vi "UpdateLoadCell.vi"(8 "Steps":i8, 9 "Address":i32, 10 "Code67Memory":refnum<k21>, 11 "Code66Memory":refnum<k21>) -> ()   [LabVIEW 2016, in "FPGAMockMDILC.lvlib"]
uses:
  FPGAMockMDILC.lvlib
  <vilib>/rvi/Emulation/niFpgaSctlEmulationGetInTimedLoop.vi
  <vilib>/Utility/error.llb/Clear Errors.vi
  <vilib>/rvi/DataTransferAndStorage/Container/Common/niFpgaContainerExecOnDevCompGetState.vi
  <vilib>/rvi/Emulation/niFpgaEmulationIsFPGAContextNoSignature.vi
  <vilib>/rvi/DataTransferAndStorage/Container/Common/niFpgaContainerGetUniqueNameForEmu.vi
  <vilib>/rvi/Emulation/niFpgaProcessEmulError.vi
  <vilib>/rvi/errors/nirviReportUnexpectedCaseInternalError (U32).vi
  <vilib>/rvi/Memory/Memory_Emulation/niFpgaMemoryEmulationCacheClearOnFirstRun.vi
  <vilib>/rvi/Memory/Memory_Emulation/nirvimemoryEmulationManagerCache_MakeExclusive.vi
  <vilib>/rvi/Memory/Memory_Emulation/niFpgaMemoryEmulationValidateCache.vi
  <vilib>/rvi/Memory/Memory_Emulation/nirvimemoryEmulationManagerCache_InsertValue.vi
  <vilib>/rvi/Memory/Memory_Emulation/nirvimemoryEmulationManagerCache_ReleaseExclusive.vi
  <vilib>/rvi/Memory/Memory_Emulation/nirvimemoryEmulationManagerCache_GetValue.vi
  <vilib>/rvi/Memory/Memory_Emulation/nirvimemoryEmulationManagerCache_SetValue.vi
  <vilib>/rvi/Emulation/niFpgaSctlEmulationResourceMgr.vi
  <vilib>/rvi/DataTransferAndStorage/Container/XNode/niFpgaContainer.xnode
  <vilib>/rvi/Memory/Memory_Emulation/niFpgaMemoryEmulationRefIn.vi
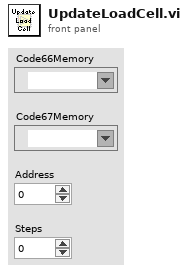
[diagram p1: front panel]
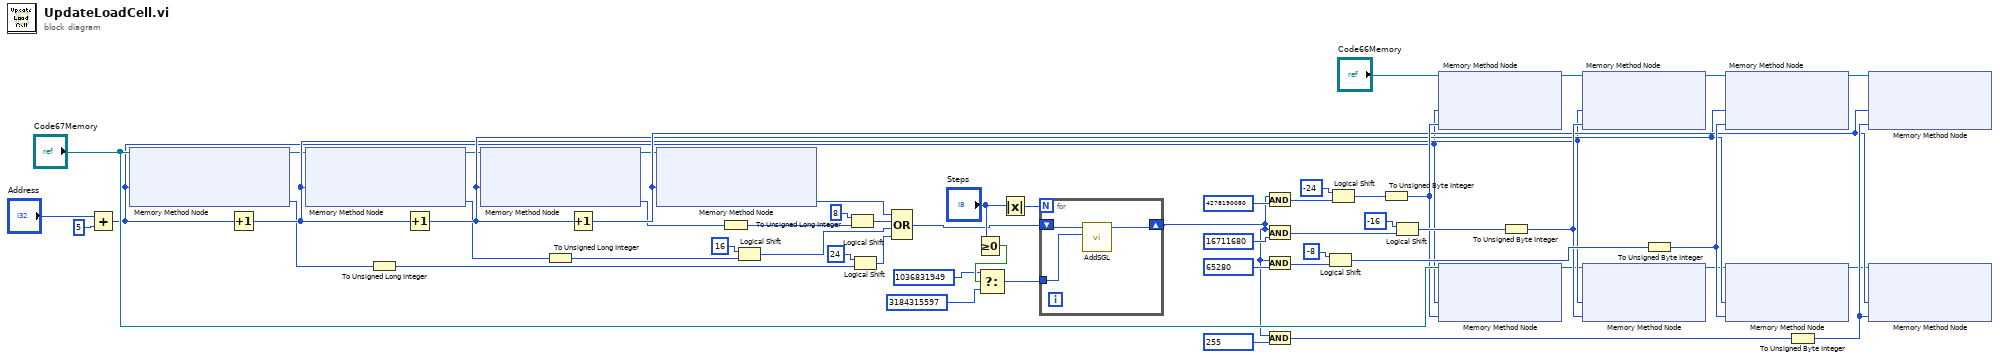
[diagram p0: block diagram]
diagram:
  n1 = Add(x="Address", y=5) -> (x+y=w41:i32)
  n2 = xnode ("Memory Method Node")("Address"=w41, "Memory In"="Code67Memory") -> ("Data"=w12:u8, "Memory Out"=w9:refnum<k21>)
  n3 = Increment(x=w41) -> (x+1=w43:i32)
  n4 = xnode ("Memory Method Node")("Address"=w43, "Memory In"=w9) -> ("Data"=w17:u8, "Memory Out"=w21:refnum<k21>)
  n5 = To Unsigned Long Integer(number=w12) -> (unsigned 32bit integer=w13:u32)
  n6 = Increment(x=w43) -> (x+1=w45:i32)
  n7 = xnode ("Memory Method Node")("Address"=w45, "Memory In"=w21) -> ("Data"=w20:u8, "Memory Out"=w22:refnum<k21>)
  n8 = To Unsigned Long Integer(number=w17) -> (unsigned 32bit integer=w16:u32)
  n9 = Increment(x=w45) -> (x+1=w47:i32)
  n10 = xnode ("Memory Method Node")("Address"=w47, "Memory In"=w22) -> ("Data"=w26:u8)  [unwired: 1 out]
  n11 = To Unsigned Long Integer(number=w20) -> (unsigned 32bit integer=w18:u32)
  n12 = Logical Shift(y=i16 16, x=w16) -> (x << y=w24:u32)
  n13 = Logical Shift(y=i16 8, x=w18) -> (x << y=w25:u32)
  n14 = Logical Shift(y=i16 24, x=w13) -> (x << y=w23:u32)
  n15 = Compound Arithmetic op=OR(w26, w25, w24, w23) -> (w2:u32)
  n16 = Greater Or Equal To 0?(x="Steps") -> (x >= 0?=w6:bool)
  n17 = Select(t=u32 1036831949, s=w6, f=u32 3184315597) -> (s? t:f=w3:u32)
  n18 = Absolute Value(x="Steps") -> (abs(x)=w8:i8)
  n19 = for {
    N: w8 -> [_]
    tunnel: w3 -> [w59]
    shift-right: [w57] -> w1
    shift-left: w2 -> [w58]
    n20 = call "AddSGL.vi"("Y"=w59, "X"=w58) -> ("Output"=w57:u32)  [unwired: 9 in]
  }
  n21 = And(x=w1, y=u32 4278190080) -> (x .and. y?=w31:u32)
  n22 = And(x=w1, y=u32 16711680) -> (x .and. y?=w32:u32)
  n23 = And(x=w1, y=u32 65280) -> (x .and. y?=w33:u32)
  n24 = And(x=w1, y=u32 255) -> (x .and. y?=w48:u32)
  n25 = Logical Shift(y=i16 -8, x=w33) -> (x << y=w54:u32)
  n26 = Logical Shift(y=i16 -24, x=w31) -> (x << y=w50:u32)
  n27 = To Unsigned Byte Integer(number=w50) -> (unsigned 8bit integer=w51:u8)
  n28 = Logical Shift(y=i16 -16, x=w32) -> (x << y=w52:u32)
  n29 = xnode ("Memory Method Node")("Address"=w41, "Data"=w51, "Memory In"="Code66Memory") -> ("Memory Out"=w38:refnum<k21>)
  n30 = xnode ("Memory Method Node")("Address"=w41, "Data"=w51, "Memory In"="Code67Memory") -> ("Memory Out"=w42:refnum<k21>)
  n31 = To Unsigned Byte Integer(number=w52) -> (unsigned 8bit integer=w53:u8)
  n32 = xnode ("Memory Method Node")("Address"=w43, "Data"=w53, "Memory In"=w38) -> ("Memory Out"=w39:refnum<k21>)
  n33 = xnode ("Memory Method Node")("Address"=w43, "Data"=w53, "Memory In"=w42) -> ("Memory Out"=w44:refnum<k21>)
  n34 = To Unsigned Byte Integer(number=w54) -> (unsigned 8bit integer=w55:u8)
  n35 = xnode ("Memory Method Node")("Address"=w45, "Data"=w55, "Memory In"=w39) -> ("Memory Out"=w40:refnum<k21>)
  n36 = xnode ("Memory Method Node")("Address"=w45, "Data"=w55, "Memory In"=w44) -> ("Memory Out"=w46:refnum<k21>)
  n37 = To Unsigned Byte Integer(number=w48) -> (unsigned 8bit integer=w49:u8)
  n38 = xnode ("Memory Method Node")("Address"=w47, "Data"=w49, "Memory In"=w40) -> ()  [unwired: 1 out]
  n39 = xnode ("Memory Method Node")("Address"=w47, "Data"=w49, "Memory In"=w46) -> ()  [unwired: 1 out]
